vi "GDSLvLib_StoreLibType.vi"(0 "Lib Refnum In":refnum<vi>, 1 "LibSettings":T1, 3 "CheckAndFixConnectorPaneType(False)":bool, 5 "error in (no error)":errorcluster) -> (14 "Lib Refnum Out":refnum<vi>, 19 "error out":errorcluster)   [LabVIEW 2014]
uses:
  <resource>/Framework/Providers/Open_GDS/ClassProviders/Common/LvLib_class/GDSLvLib_LibSettingsType.ctl
  <resource>/Framework/Providers/Open_GDS/ClassProviders/Common/LvClass_class/GDSLvClass_PlugIn.ctl
  <resource>/Framework/Providers/Open_GDS/ClassProviders/Common/LvClass_class/GDSLvClass_PlugInTypes.ctl
  <resource>/Framework/Providers/Open_GDS/ClassProviders/Common/LvLib_class/GDSLvLib_LibTypeSettingNames.ctl
  <resource>/Framework/Providers/Open_GDS/ClassProviders/Common/ScriptingFunctions/Scripting_ConnectorPanePatternType.ctl
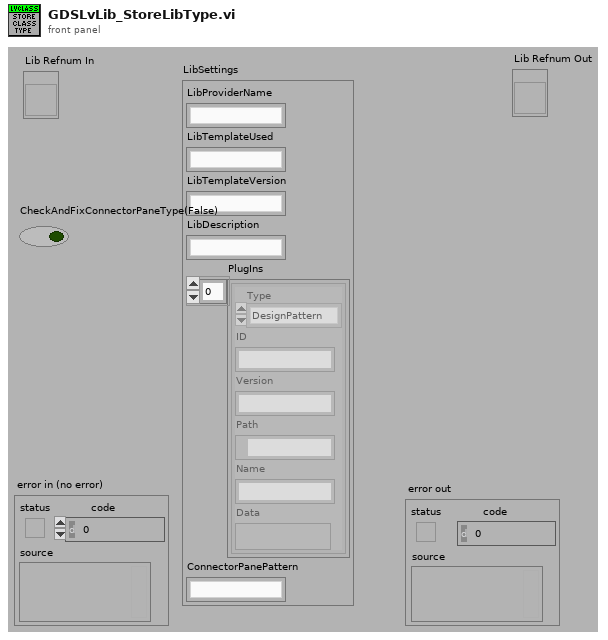
[diagram p1: front panel]
types:
  T1 = typedef "GDSLvLib_LibSettingsType.ctl" = cluster{"LibProviderName":string, "LibTemplateUsed":string, "LibTemplateVersion":string, "LibDescription":string, "PlugIns":T2[], "ConnectorPanePattern":string}
  T2 = typedef "GDSLvClass_PlugIn.ctl" = cluster{"Type":T3, "ID":string, "Version":string, "Path":path, "Name":string, "Data":variant}
  T3 = typedef "GDSLvClass_PlugInTypes.ctl" = enum16{"DesignPattern", "MethodTypes"}
  T4 = typedef "GDSLvLib_LibTypeSettingNames.ctl" = enum16{"EndevoGOOP_LibProvider", "EndevoGOOP_TemplateUsed", "EndevoGOOP_TemplateVersion", "EndevoGOOP_PlugIns", "EndevoGOOP_ConnectorPanePattern"}
  T5 = typedef "Scripting_ConnectorPanePatternType.ctl" = u16
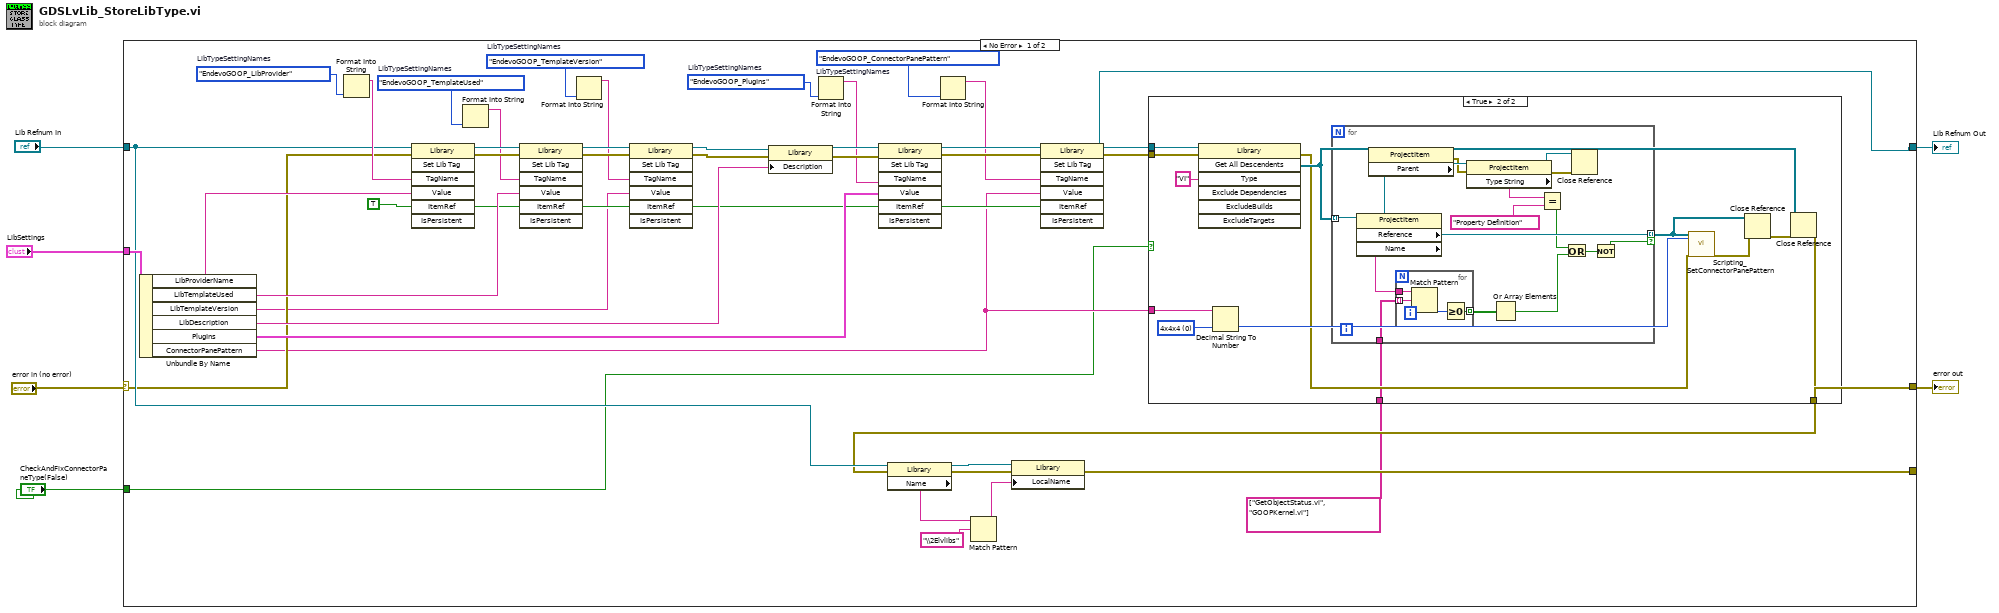
[diagram p0: block diagram]
diagram:
  n1 = case shown="No Error" "error in (no error)" {
    selector: "error in (no error)" -> [w25 w83]
    tunnel: [w15 w83] -> w5
    tunnel: "Lib Refnum In" -> [w26 w82]
    tunnel: [w13 w82] -> w3
    tunnel: "LibSettings" -> [w38 _]
    tunnel: [w18 _] -> _
    tunnel: "CheckAndFixConnectorPaneType(False)" -> [w14 _]
    frame No Error {
      w7 = GDSLvLib_LibTypeSettingNames."EndevoGOOP_ConnectorPanePattern"  # LibTypeSettingNames
      w8 = GDSLvLib_LibTypeSettingNames."EndevoGOOP_PlugIns"  # LibTypeSettingNames
      w9 = GDSLvLib_LibTypeSettingNames."EndevoGOOP_TemplateVersion"  # LibTypeSettingNames
      w10 = GDSLvLib_LibTypeSettingNames."EndevoGOOP_TemplateUsed"  # LibTypeSettingNames
      w11 = GDSLvLib_LibTypeSettingNames."EndevoGOOP_LibProvider"  # LibTypeSettingNames
      w27 = TRUE ("Is Persistent")
      n2 = Unbundle By Name(w38) -> ("LibProviderName"=w37:string, "LibTemplateUsed"=w36:string, "LibTemplateVersion"=w24:string, "LibDescription"=w35:string, "PlugIns"=w32:T2[], "ConnectorPanePattern"=w17:string)
      n3 = Format Into String(w11) -> (resulting string=w41:string)  [unwired: 3 in, 1 out]
      n4 = invoke class="Library" method="Set Lib Tag"(reference=w26, error in=w25, "TagName"=w41, "Value"=w37, "ItemRef"=w27) -> (reference out=w47:refnum<vi>, error out=w46:errorcluster)  [unwired: 2 in, 5 out]
      n5 = Format Into String(w10) -> (resulting string=w40:string)  [unwired: 3 in, 1 out]
      n6 = invoke class="Library" method="Set Lib Tag"(reference=w47, error in=w46, "TagName"=w40, "Value"=w36, "ItemRef"=w27) -> (reference out=w45:refnum<vi>, error out=w44:errorcluster)  [unwired: 2 in, 5 out]
      n7 = Format Into String(w9) -> (resulting string=w39:string)  [unwired: 3 in, 1 out]
      n8 = invoke class="Library" method="Set Lib Tag"(reference=w45, error in=w44, "TagName"=w39, "Value"=w24, "ItemRef"=w27) -> (reference out=w43:refnum<vi>, error out=w42:errorcluster)  [unwired: 2 in, 5 out]
      n9 = property class="Library"(reference=w43, error in=w42, "Description"=w35) -> (reference out=w34:refnum<vi>, error out=w33:errorcluster)
      n10 = Format Into String(w8) -> (resulting string=w31:string)  [unwired: 3 in, 1 out]
      n11 = invoke class="Library" method="Set Lib Tag"(reference=w34, error in=w33, "TagName"=w31, "Value"=w32, "ItemRef"=w27) -> (reference out=w30:refnum<vi>, error out=w29:errorcluster)  [unwired: 2 in, 5 out]
      n12 = Format Into String(w7) -> (resulting string=w28:string)  [unwired: 3 in, 1 out]
      n13 = invoke class="Library" method="Set Lib Tag"(reference=w30, error in=w29, "TagName"=w28, "Value"=w17, "ItemRef"=w27) -> (reference out=w13:refnum<vi>, error out=w16:errorcluster)  [unwired: 2 in, 5 out]
      n14 = case shown="True" w14 {
        tunnel: w13 -> [_ w61]
        tunnel: w17 -> [_ w59]
        tunnel: w16 -> [w48 w52]
        tunnel: [w48 w50] -> w15
        tunnel: string[] ["GetObjectStatus.vi", "GOOPKernel.vi"] -> [_ w49]
        frame False {
        }
        frame True {
          w58 = T5 0 items=["4x4x4", "5x6x5", "6x8x6"] ("Pattern")
          n15 = invoke class="Library" method="Get All Descendents"(reference=w61, error in=w52, "Type"="VI") -> (error out=w51:errorcluster, "All Descendents"=w53:refnum<vi>[])  [unwired: 4 in, 5 out]
          n16 = Decimal String To Number(string=w59, default (0L)=w58) -> (number=w57:u16)  [unwired: 1 in, 1 out]
          n17 = for {
            tunnel: w53 -> [w77] mode=indexing
            tunnel: [w72] -> w56 mode=indexing if=w73
            tunnel: w49 -> [w75]
            n18 = property class="ProjectItem"(reference=w77) -> (reference out=w71:refnum<vi>, "Reference"=w72:refnum<vi>, "Name"=w76:string)  [unwired: 1 in, 1 out]
            n19 = property class="ProjectItem"(reference=w71) -> (error out=w62:errorcluster, "Parent"=w70:refnum<vi>)  [unwired: 1 in, 1 out]
            n20 = for {
              tunnel: w76 -> [w81]
              tunnel: w75 -> [w80] mode=indexing
              tunnel: [w78] -> w74 mode=indexing
              n21 = Match Pattern(string=w81, regular expression=w80) -> (offset past match=w79:i32)  [unwired: 1 in, 3 out]
              n22 = Greater Or Equal To 0?(x=w79) -> (x >= 0?=w78:bool)
            }
            n23 = property class="ProjectItem"(reference=w70, error in=w62) -> (reference out=w64:refnum<vi>, error out=w63:errorcluster, "Type String"=w69:string)
            n24 = Or Array Elements(Boolean array=w74) -> (logical OR=w66:bool)
            n25 = Equal?(x=w69, y="Property Definition") -> (x = y?=w67:bool)
            n26 = Or(x=w67, y=w66) -> (x .or. y?=w65:bool)
            n27 = Close Reference(reference=w64, error in (no error)=w63) -> ()  [unwired: 1 out]
            n28 = Not(x=w65) -> (.not. x?=w73:bool)
          }
          n29 = call <resource>:"Scripting_SetConnectorPanePattern.vi"("VIPath(s)/ViRef(s)"=w56, "Pattern"=w57, "error in (no error)"=w51) -> ("error out"=w55:errorcluster)  [unwired: 16 in]
          n30 = Close Reference(reference=w56, error in (no error)=w55) -> (error out=w54:errorcluster)
          n31 = Close Reference(reference=w53, error in (no error)=w54) -> (error out=w50:errorcluster)
        }
      }
      n32 = property class="Library"(reference=w26, error in=w15) -> (reference out=w23:refnum<vi>, error out=w22:errorcluster, "Name"=w21:string)
      n33 = Match Pattern(string=w21, regular expression="\\2Elvlibs") -> (before substring=w19:string)  [unwired: 1 in, 3 out]
      n34 = property class="Library"(reference=w23, error in=w22, "LocalName"=w19) -> (error out=w18:errorcluster)  [unwired: 1 out]
    }
    frame Error {
    }
  }
  "Lib Refnum Out" <- w3
  "error out" <- w5
